vi "Main_08B_Long Wait.vi"() -> ()   [LabVIEW 2025]
uses:
  Cluster_3D Pos.ctl
  41698488-36b5-4046-9fd7-0d51cedffe47.vi
  2bdc9d8d-ae33-491b-9533-2d130997e3b1.vi
  Utility/Universal Utility/TypeDefs_Utility/Cluster_Row-Column.ctl
  9e3f57c0-2ef8-4495-8287-c6a42a5fb955.vi
  Utility/Universal Utility/TypeDefs_Utility/ENUM_4 Directions U-D-L-R.ctl
  Utility/Universal Utility/TypeDefs_Utility/ENUM_8 Directions U-D-L-R.ctl
panel:
  out "Cluster Out":cluster{"Numeric":dbl, "3D Pos":T1, "3D Pos":T1}
  out "Target":i32
  out "Last Size":i32
  out "Numeric":i32
  out "x-y 2":i32
  out "size(s)":i32
  out "x-y":i32
  out "map":map{T1, set{T1}}(c390)
  out "Distances":T2(array[cluster])
  in  "3D Pos":T1
  out "MATCH":bool
  in  "Select Data":enum32{"Example", "Puzzle"}(tab)
  in  "EX Target":u64=25272
  in  "Example":string="162,817,812\n57,618,57\n906,360,560\n592,479,940\n352,342,300\n466,668,158\n542,29,236\n431,825,988\n739,650,466\n52,470,668\n216,146,977\n819,987,18\n117,168,530\n805,96,715\n346,949,466\n970,615,88\n941,993,340\n862,61,35\n984,92,344\n425,690,689"
  in  "Puzzle":string="93612,76992,69452\n4387,60049,8877\n43126,39737,84757\n30167,68987,19789\n92427,53000,95237\n38193,19273,23561\n54992,34511,43980\n11107,44787,52686\n35724,98740,19812\n28016,57751,86155\n93461,77703,78395\n94606,79586,97929\n67878,92289,42528\n38971,54378,98204\n66002,25958,89347\n40281,30990,67294\n25898,31190,14029\n85535,48773,26872\n10128,70597,46452\n68618,23612,85624\n79490,1682,569\n8828,51411,60251\n38583,16324,14091\n10437,63697,61596\n56370,26228,17029\n86199,8063,16493\n20471,66847,99889\n28748,63929,18749\n19248,83995,67615\n333,91140,79303\n59093,5932,49628\n65463,73678,60286\n87559,27061,41247\n424,28274,74202\n85572,19477,32761\n88116,2580,65047\n77302,37669,40015\n7664,30793,17676\n7152,87786,56278\n21754,53651,91511\n19205,97579,71254\n13841,24770,87922\n60676,26132,30482\n10161,34169,42397\n97588,95253,77422\n62674,99068,96065\n3701,85077,92763\n87646,99624,9786\n79480,48455,82469\n85485,88400,12789\n80002,63227,89969\n78922,68131,54845\n11326,3980,91289\n37613,85718,1487\n73551,87391,77749\n18494,53007,56937\n95754,20192,31376\n81009,94209,66866\n89029,86481,28533\n73124,31585,3562\n5647,86375,87389\n17667,62606,81057\n90251,13392,46704\n8922,53813,49554\n90818,72498,63116\n63706,12205,48645\n86075,45959,79136\n8533,98522,94830\n13261,87807,47571\n85512,34571,10686\n70830,45794,26572\n70838,85387,63507\n50514,2902,47654\n97257,76204,25909\n20663,49002,12395\n14787,22089,91493\n9519,20986,37182\n48407,1747,57434\n84550,61928,41891\n27065,7926,77657\n32551,75407,17933\n44728,48491,5096\n28667,99071,90157\n98892,74499,37947\n75619,55121,72752\n36135,20145,68562\n33258,19964,28963\n66217,41845,39708\n32152,82331,42510\n38241,71629,84071\n63645,42508,41998\n18010,23872,31891\n30919,69353,79552\n5249,74361,18723\n51253,57096,69531\n54551,72707,27442\n87816,89043,21120\n43115,24297,19479\n10017,68608,64216\n38916,98813,18429\n53460,96455,10528\n1528,25204,29747\n59806,11528,62206\n84940,6921,98186\n55,22445,44444\n48901,95321,2434\n36897,31163,71124\n733,10092,43971\n95769,23499,86894\n58488,65824,44700\n95535,95053,28430\n62042,11824,48380\n47371,59378,9083\n87851,59391,33276\n71416,91746,80466\n20986,14005,28560\n62877,91310,56300\n44999,12630,89580\n12814,17342,311\n75884,25052,43459\n17057,50968,25293\n8779,78959,17492\n37260,26515,88716\n93030,14321,95804\n51240,43987,47003\n19716,71779,92039\n38192,96721,59996\n3751,16201,26085\n23562,83044,98517\n21091,69932,70564\n17906,89206,87817\n15112,8697,39582\n50853,23583,25901\n4031,58523,46946\n29574,85339,94502\n2159,28840,67804\n64232,21352,6079\n69968,53511,19694\n64707,83228,92602\n68033,91486,5930\n88327,83351,44501\n48616,4913,23373\n64394,88985,96012\n7137,22829,95789\n61147,23131,27577\n9220,73362,24735\n77484,65386,87676\n19406,27628,27294\n36096,5448,80101\n41415,71615,96750\n49579,73718,75680\n51667,75635,2150\n58588,13959,21674\n3301,85861,9573\n39663,82812,63976\n77881,12060,64325\n32096,56047,49426\n87020,81590,63482\n11350,22612,68794\n34318,87015,28581\n88333,30415,72842\n14284,31669,98394\n91299,33003,98512\n50558,25664,87891\n45463,92120,88896\n78928,17342,53217\n85152,36483,90933\n32494,63948,13733\n79538,15123,59524\n13272,69237,88883\n71440,34646,36000\n70887,92196,70756\n86682,49869,59461\n87014,69218,96246\n85096,62446,58342\n47656,42067,94693\n76389,21187,19854\n98808,95119,66355\n56317,4067,58089\n62979,31016,54595\n95574,94910,44555\n92818,89957,30178\n88205,83421,11231\n98025,26158,67351\n34996,37782,12656\n7275,92020,69192\n61755,48578,74891\n91077,87591,13567\n47178,98753,67298\n24890,185,41055\n21656,10424,76098\n36907,5392,33161\n1196,87844,89911\n62084,33566,56665\n66936,13949,44242\n10287,7906,50612\n94242,25001,57410\n75412,1024,29512\n90851,87543,72388\n71747,19001,91980\n22967,72331,12208\n29687,34581,5318\n52323,58423,16852\n86287,3765,36953\n15503,61881,49607\n17730,83252,72329\n32791,46945,9909\n90377,15005,82108\n25088,43430,50889\n30937,67449,69570\n27055,70369,20047\n87796,33912,38981\n61308,25361,93385\n92140,77658,13928\n22619,38036,36441\n66615,58337,19579\n69481,81387,29719\n96348,68719,86050\n50514,639,29192\n75973,520,69761\n82361,79014,99108\n84447,68240,70851\n1603,1169,79818\n17505,5417,49001\n42348,26283,64808\n53052,35593,79353\n29059,44086,34246\n19705,32222,54841\n93505,73226,37229\n88280,88881,65243\n31982,61769,85501\n18942,69659,87848\n48747,77115,64412\n89986,59345,39585\n92036,77473,89017\n54927,93308,13866\n62414,96971,46218\n18054,44880,20543\n18191,85757,79281\n55277,56892,25137\n56722,15970,49886\n65888,61906,88954\n21214,43085,32786\n79619,24041,30679\n22962,60563,90448\n24703,43433,54346\n64964,61426,85237\n81713,50846,23776\n16354,44817,55696\n2131,92987,36071\n24669,58903,97840\n34050,79236,15174\n94757,87186,41770\n60958,81684,89389\n70618,56638,1431\n15922,77068,73670\n84295,36683,59806\n39229,8110,32311\n9957,37073,62331\n58126,91378,50095\n43938,84938,37934\n46924,27412,73996\n78529,43275,80069\n47252,68636,49729\n11419,1422,86133\n32065,82752,94710\n21983,2625,75459\n44369,40437,65291\n45830,99247,97279\n102,35695,58176\n31421,83303,74978\n58281,98901,45492\n106,49263,7938\n14420,24582,44323\n68568,24062,71612\n16050,65447,90641\n7423,8218,42238\n16769,75102,10654\n91505,32646,7194\n94158,35310,78925\n8512,2585,65102\n78362,24338,27827\n61073,96429,1483\n55466,2563,6915\n76849,20355,4244\n23720,88978,85697\n4881,40227,59389\n90297,3954,2223\n71850,58017,89245\n88343,36437,43379\n48699,55848,41462\n87085,80923,41276\n8190,65515,49515\n60930,91345,56495\n775,157,41546\n78449,37056,92044\n25226,37026,8384\n83556,2712,79328\n23265,52246,97851\n84479,51110,40981\n62886,35622,78961\n6523,92713,24122\n25314,54911,73916\n35030,4968,50659\n49041,83519,77623\n15167,26960,96355\n16247,64185,99408\n18474,61281,4969\n13926,31813,16094\n15725,68810,87796\n15464,46735,8813\n13805,10520,11814\n16255,71827,53917\n17481,74068,39973\n1780,6131,70717\n96873,33332,58634\n75700,9121,4357\n15100,24737,23182\n21595,73141,60112\n17623,46752,17930\n966,77550,1372\n23916,5486,61016\n58073,54435,99676\n63398,25454,22034\n11040,78676,89673\n72346,68534,60847\n86865,20480,28605\n10868,89008,17327\n9838,37312,78948\n9843,72664,46882\n25362,3537,55029\n25124,98455,46040\n67429,30617,65289\n50349,91411,86860\n88161,26971,2438\n55654,9333,21695\n21824,81354,24579\n74930,71845,25730\n31018,58510,74464\n63758,31045,74703\n66762,78487,4118\n51908,57077,1574\n36829,63414,74887\n70493,64836,64929\n67420,65219,8818\n67566,17153,99697\n31824,74123,30207\n56502,53943,35115\n17246,97907,98834\n68705,29666,71246\n27724,15999,56550\n60276,22366,14653\n46389,53387,87116\n3235,14486,91436\n49732,63892,87340\n87008,94331,58514\n32145,38609,71845\n64572,18666,90042\n12352,11171,65795\n50884,39309,7436\n72407,18819,32603\n37449,16014,50829\n50516,25437,245\n66137,40543,98203\n28102,29674,6025\n55921,37483,59917\n80575,24800,7675\n44559,17720,81000\n21868,4371,65769\n34785,60526,44642\n5726,52286,31034\n35566,72914,82787\n32070,85672,66017\n19110,93664,19934\n53538,56804,28502\n78852,78651,65871\n99691,96705,52190\n77702,9722,56604\n96505,53849,9751\n85655,28788,96526\n96697,6837,96685\n83162,25825,24329\n48579,28766,854\n88152,9279,65839\n83244,71777,64273\n67540,72397,45717\n33581,56860,73496\n41361,43101,43910\n77896,55800,6729\n11660,9790,41267\n97909,44466,33924\n75949,72557,25770\n2834,8126,65868\n9551,65106,23021\n16497,40985,62744\n2394,85493,15918\n13869,86996,34945\n7314,71681,76769\n8314,17091,51115\n21559,78084,38617\n23289,65563,77867\n56384,16752,25872\n73173,27198,18275\n14487,89322,53052\n43042,74199,19715\n79730,3967,66686\n49193,63676,8674\n75653,71020,71125\n76566,82061,60310\n62574,19011,34913\n7784,78818,4837\n96246,64285,64844\n28376,38429,5472\n29362,65551,35253\n86883,51698,98020\n24309,19686,76751\n79120,49475,86875\n21875,26909,80928\n26647,97704,47621\n81672,4744,85242\n1531,59200,59569\n32899,26845,37534\n44049,35082,85646\n76568,75911,25179\n8965,84562,95316\n84091,11217,36912\n75391,5840,53123\n65257,29963,25808\n37711,89932,64085\n58313,77455,73975\n50094,87928,18598\n5972,26111,44908\n18007,13342,78943\n76931,50984,47834\n21067,16782,67472\n15702,16241,74410\n87250,79827,72823\n39856,29885,87881\n63010,34722,55942\n66094,53196,60158\n66103,13376,41069\n50817,73301,75220\n92689,896,59366\n25127,93940,535\n26486,26180,69703\n30551,201,44121\n57951,59180,74903\n81875,39479,66376\n75608,64370,34924\n65874,46991,20843\n64546,80899,48722\n53139,81240,60912\n6408,95126,99539\n60382,32038,26842\n51897,69343,23769\n12903,64987,23678\n89816,57639,2794\n91943,17916,68132\n17058,47490,53424\n63508,59639,78981\n24149,76305,83221\n59786,97124,35477\n7654,4401,5943\n65324,87395,56976\n1254,59660,42700\n28520,51382,13607\n32395,72384,24714\n98919,51493,35815\n85861,23706,42361\n73727,19357,9192\n56244,61066,88568\n69022,93334,95441\n45135,78907,67376\n71905,21859,53682\n76240,18122,86744\n96451,36880,58724\n69809,81170,43323\n91766,30035,70211\n94430,93928,35098\n36019,86391,62142\n29610,48551,78565\n61687,61798,44674\n83243,280,87775\n12879,46004,26625\n35774,96599,27266\n54000,69437,46041\n53659,5289,64037\n74733,24414,37294\n97525,10350,59878\n27775,49801,65616\n1659,48519,9189\n4829,84196,28561\n60895,93831,21468\n61573,4274,9651\n98125,85369,35792\n52818,38024,65559\n84495,67225,93469\n32787,83707,84703\n62567,37936,64206\n94030,89183,13432\n13072,95484,27690\n23734,31846,65035\n92988,93579,66115\n78711,53315,59155\n54913,63455,29728\n62483,46401,60745\n20788,21695,50675\n42551,84909,54997\n852,73770,55668\n10942,89879,3343\n88911,85683,58125\n8888,4740,64248\n61357,52361,84989\n59211,31184,957\n68198,89759,1696\n66912,82567,26659\n63452,49304,14117\n55562,86015,61863\n96167,90245,35196\n83946,59012,8249\n83464,21575,9933\n20029,49554,45712\n45708,6745,4125\n33357,87835,35297\n86141,60426,87671\n48011,2841,34713\n70487,20646,44208\n52285,77621,30036\n59856,65624,60884\n92153,97045,59609\n77434,44541,28160\n99278,3474,2582\n44670,87341,16251\n16908,23106,9882\n3599,76235,82771\n55003,24153,14048\n31115,24573,17690\n93842,2483,76226\n19930,22308,31182\n97987,68482,5762\n97753,36572,53143\n56946,55429,42606\n4114,37864,84931\n20033,73108,2340\n63076,45812,25089\n68562,32600,71420\n60368,97785,65980\n5445,48961,97781\n58844,71797,9869\n77623,23298,19643\n68939,99057,77762\n47164,99255,46365\n17824,73903,89733\n44488,67436,26816\n10626,19619,37213\n78525,91601,18913\n87482,17097,99480\n89825,9580,23005\n81850,94513,95910\n58710,20827,82163\n84830,30431,42014\n19885,2222,91325\n29036,50455,10625\n14579,68427,88723\n46506,57905,65480\n25501,25015,65137\n34126,92382,12760\n42990,35933,69002\n76547,12396,70799\n27867,68712,54134\n58345,5062,87052\n51715,80934,28246\n74189,23723,30837\n98243,92321,40231\n42351,5969,15336\n29632,29612,22258\n31543,13513,60004\n51272,2995,7475\n96993,16572,7646\n8241,53230,7612\n20137,54640,20893\n59566,7551,18524\n40530,53994,15411\n6874,38747,96386\n60096,17731,1885\n21358,47158,57995\n48040,27043,44231\n90293,31220,5002\n87034,57231,1922\n47580,56506,51457\n21645,43851,33340\n50203,31461,99819\n29924,64669,80294\n48937,97069,87025\n56459,76682,90702\n39922,84072,64788\n56086,33603,60174\n57079,95782,95195\n93093,10317,85610\n4553,96124,53294\n70238,97923,20386\n76705,37902,51495\n18376,89053,50239\n43721,95653,31712\n97543,903,77076\n63809,98240,32449\n19598,27244,51311\n58861,93737,38995\n46246,70148,17082\n44972,2348,38868\n6647,2768,40251\n59453,62399,43434\n27211,23165,55801\n31210,4420,40809\n67954,89265,21307\n38157,58874,65993\n17047,12135,98851\n65082,3379,10087\n14995,71193,92046\n85554,218,47029\n52869,68400,61476\n15245,89469,36381\n1523,36104,35383\n81169,162,47941\n36480,61750,92719\n9137,30924,39406\n4656,6959,26256\n94128,50715,27623\n17165,55297,17490\n93520,76418,8404\n31533,5640,75764\n3115,47128,2667\n70908,20297,33409\n91667,83564,10987\n78738,79975,79614\n98601,79197,63374\n22489,6709,19769\n3661,48606,4034\n62587,69293,92052\n31430,11646,58643\n80493,23478,52020\n76806,36625,61325\n52254,77479,79176\n89958,48556,1961\n5928,19241,90408\n71968,16233,65908\n49587,3396,51724\n15836,73105,68814\n87142,20107,78921\n19987,26258,32877\n47137,5614,19848\n88710,50130,58513\n12385,24867,62286\n88852,6913,44817\n21656,66145,71816\n13390,54530,54277\n557,41725,27372\n30345,90380,49797\n95541,28277,63610\n15296,61358,32017\n96483,11065,83679\n31183,4570,40265\n69674,28710,2052\n21841,48430,57641\n20947,65038,17338\n39281,94409,83606\n53035,53090,82421\n22343,46641,9487\n37999,11874,10825\n28891,74850,94585\n87115,56628,33382\n14619,74286,45544\n39133,78470,91243\n42199,76781,37404\n64919,33295,42593\n37280,99390,75546\n99850,21071,86687\n12561,14737,51205\n82463,8628,46379\n66413,6177,22765\n64129,76197,71439\n42257,60362,76910\n88537,67489,68630\n38,59181,27553\n18122,55369,49886\n36309,97303,40682\n51847,12862,36119\n63247,24005,69216\n79104,66384,54736\n56017,25641,12457\n44064,88259,80773\n29737,522,94568\n45720,48619,8513\n32824,94363,98444\n66637,42496,26435\n2012,34374,99911\n63462,34544,82946\n60906,96191,27861\n889,8875,96367\n20701,850,32374\n48614,31194,51795\n81219,24377,57375\n80635,53805,27351\n73080,55463,50428\n63827,57808,55144\n51107,90419,84912\n18717,94186,31613\n49169,44719,10443\n39615,75279,12347\n11964,45685,47665\n30923,15472,65080\n5,94188,54596\n14379,13017,44646\n77743,60302,80107\n9067,49328,81390\n3402,88018,48284\n8590,94702,4002\n53713,46872,45856\n88918,2415,28532\n46287,21781,14851\n29324,9071,81874\n96983,92983,94390\n26328,6604,67828\n15607,19849,9427\n3777,80212,69260\n66785,89681,58809\n47599,81474,12698\n19680,28606,58721\n84565,96029,9266\n6807,28162,25245\n37858,37187,33146\n74215,20317,21602\n36577,27799,76382\n7377,35371,6580\n7134,79656,97584\n9214,10648,27402\n71686,59728,6298\n19675,43121,23335\n59814,19764,9046\n29503,20036,61270\n21728,78643,8960\n25275,32799,80768\n44283,98410,81536\n79332,8520,54150\n45424,1453,21479\n94250,78055,73228\n79489,63243,23534\n74398,21497,19692\n26191,34756,90513\n15902,65731,1896\n20962,19514,89850\n19048,85210,61442\n95612,27282,33774\n34539,17019,59356\n15886,4956,6561\n85554,43774,56068\n83399,44069,83268\n24967,47996,80688\n4261,39672,3487\n1927,90969,36407\n56341,31181,98469\n59463,4377,44429\n98081,89435,28196\n47337,146,41069\n34676,62991,93667\n40830,18095,3895\n33969,71800,98522\n55019,22833,33982\n18690,49810,11880\n49895,63070,57918\n65670,75982,47329\n86680,2893,7573\n5834,19741,15335\n84314,61210,54625\n38876,95177,55552\n93526,89293,47002\n17120,25610,64975\n86677,14247,90832\n22687,49968,65263\n33489,61528,47384\n24128,84568,80402\n32790,66977,67469\n31024,33923,53791\n70747,28366,81550\n50357,79826,64276\n19955,61357,45034\n76265,15144,70455\n33272,27568,76909\n84054,28474,14905\n81452,3560,64204\n2995,78946,98322\n56789,88645,28228\n55217,64868,79116\n53070,48551,745\n68657,22409,8500\n19161,61390,32918\n90698,82905,97853\n5723,32433,63684\n34840,90469,60825\n56921,24222,16744\n29618,35579,65053\n13778,57959,19521\n25635,79962,26765\n11711,67792,70774\n25724,32520,56341\n60970,2201,40013\n12431,49332,27831\n42375,12958,13514\n370,13074,49841\n91947,38771,98238\n26114,98967,4911\n36520,71551,49807\n12961,85927,32810\n41687,29135,297\n13647,65415,53114\n14884,74124,94717\n55608,71741,17940\n93046,29518,14342\n74408,38008,7480\n28472,49579,78045\n30644,35566,90190\n1309,18579,30254\n97408,9395,71712\n37963,73038,17907\n9746,1554,53649\n17312,72556,34581\n30416,98565,14025\n67271,28750,53687\n89089,94797,85638\n5584,98314,42396\n27573,12427,67217\n9685,20315,45779\n5783,89296,50119\n7395,30,59651\n59962,33958,16528\n86075,23394,31491\n63546,81157,1594\n79123,11575,47557\n18756,75540,70443\n72748,68961,58742\n81525,73484,89742\n21011,49906,40935\n73943,81252,41073\n70776,51604,32224\n80561,65802,5922\n51505,27172,13520\n26382,9698,48756\n2966,37811,41624\n64790,93568,62536\n11099,33411,14293\n82091,74600,4338\n65085,60858,10082\n10035,21650,50785\n63805,33377,24475\n21382,39590,34505\n97345,3372,97760\n70419,80414,3046\n69513,27185,34584\n45800,92516,45439\n35481,65400,79823\n29374,6114,11941\n14303,82901,68795\n41717,69307,75349\n56279,66633,83524\n1428,66470,56206\n12553,6733,20622\n86659,41648,61379\n52033,36683,50080\n86318,10074,13631\n45812,45986,76341\n15567,44527,88436\n8379,59777,5722\n32237,18036,35978\n93679,5115,61935\n29374,36888,40254\n40168,44291,77176\n35156,24957,90910\n41864,98051,46439\n55645,27893,16675\n59670,98073,46841\n22314,81305,24733\n61273,22761,81192\n11266,14830,95245\n22284,40607,66310\n64598,79802,15581\n28610,12550,19851\n91295,60386,36743\n49527,66039,86751\n88255,50623,11696\n36872,95176,1262\n16382,84203,28357\n62874,36513,89144\n80390,41087,3818\n28934,77608,84891\n50028,68867,41659\n97663,86772,45290\n17334,17423,10170\n86813,9459,20678\n7354,26123,3088\n34601,83872,75235\n82487,85716,87179\n74872,55822,94773\n67775,20758,74726\n1637,23257,96839\n70086,38606,11329\n37333,4381,74577\n96787,23125,65361\n16240,10806,28282\n45777,86620,58681\n36901,96007,61808\n59798,96493,52712\n14613,28066,56986\n22873,73388,8548\n83152,66623,6706\n89253,53707,70248\n63732,55857,79585\n33389,99411,36126\n30138,88565,73193\n33385,56862,9781\n79007,32407,2149\n20654,78581,52328\n45915,25675,21594\n7534,54164,58394\n33997,15513,56367\n84919,21671,57105\n64175,41950,67051\n24936,26061,83072\n35451,62404,35874\n88295,14526,66310\n51289,61271,70041\n67716,12185,49570\n93006,31081,47748\n48016,50057,50060\n6631,7960,36378\n78124,51652,45315\n84586,11610,77166\n59601,95521,21125\n38937,84911,35085\n39499,37095,46732\n93972,71312,67295\n8864,15288,17706\n23399,15100,53520\n72344,82783,41899\n45766,36673,75853\n19760,87756,29939\n25227,74446,3738\n14331,10331,24476\n76223,50493,23898\n18356,62271,85875\n53608,20015,32714\n83392,67440,55013\n68424,46958,45601\n19431,26823,16321\n38932,60197,69781\n40297,68548,88034\n2968,29193,15002\n92059,26056,54737\n54184,66310,1075\n95784,57910,81595\n75602,59936,8544\n72249,27430,48332\n55862,41522,43934\n414,95763,96341\n33017,8463,42855\n51476,85018,43369\n60252,91356,87437\n36938,80351,62343\n84358,62436,51394\n88131,91800,50091\n75336,70492,41687\n91456,89983,51215\n17937,73395,45724\n80843,13138,64230\n49657,60368,32741\n56682,33989,9564\n73621,44474,4935\n63853,84785,75892\n29391,81042,4538\n31349,63646,21745\n55645,20057,48322\n51551,58220,79615\n21562,48950,99930\n1841,5768,17379\n40557,47811,27557\n20849,49275,68348\n44177,45015,99771\n15266,88740,35835\n22445,30430,59975\n68881,21591,89341\n76719,38478,66227\n73301,82485,38111\n8828,57991,18536\n94665,49942,59110\n15225,58083,66890\n29518,68804,75755\n50130,82904,45313\n63183,52674,91427\n97487,63178,89472\n3968,12975,47549\n22818,54619,79778"
  in  "Puzzle Target":u64=3767453340
  out "Answer":u64
  # "18446744073182037660 Is Too HIGH"
  # "15980 Too LOW"
  # "Product of the X Positions that connected\nall boxes"
  # "Product of the X Positions that connected\nall boxes"
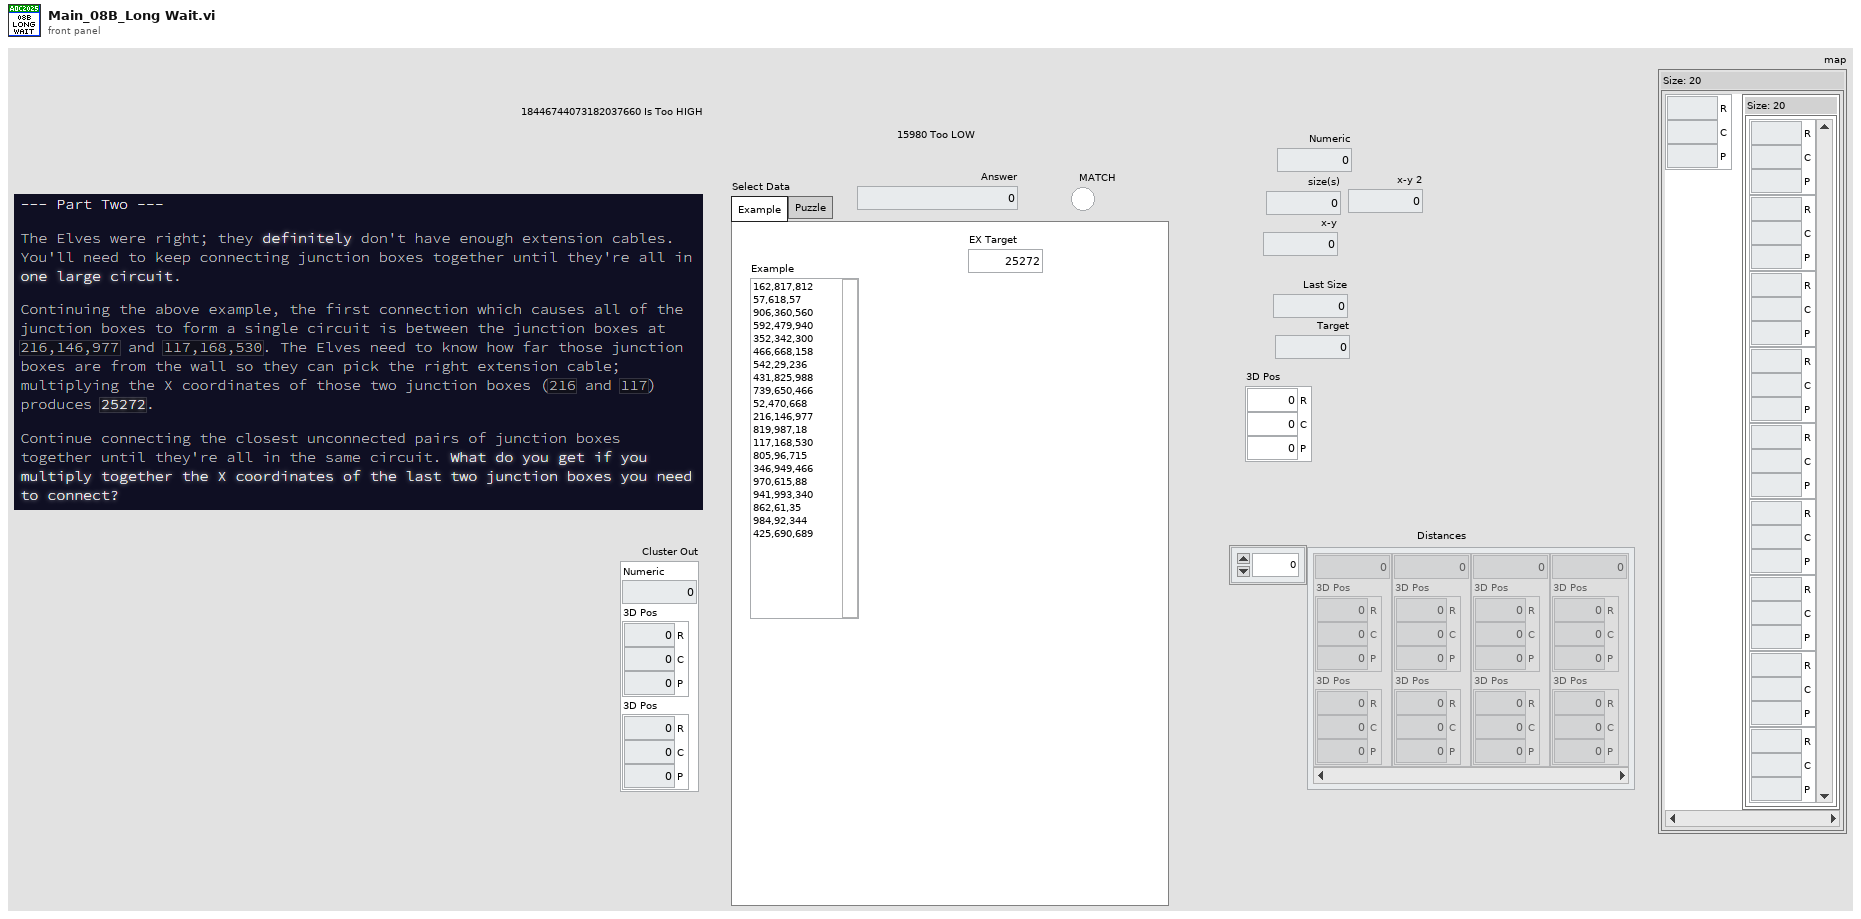
[diagram p1: front panel]
types:
  T1 = typedef "Cluster_3D Pos.ctl" = cluster{"R":i32, "C":i32, "P":i32}
  T2 = cluster{"Numeric":dbl, "3D Pos":T1, "3D Pos":T1}[]
  T3 = typedef "ENUM_8 Directions U-D-L-R.ctl" = enum16{"Up;-1,0", "Up-Right;-1,1", "Right;0,1", "Down-Right;1,1", "Down;1,0", "Down-Left;1,-1", "Left;0,-1", "Up-Left;-1,-1"}
  T4 = typedef "ENUM_4 Directions U-D-L-R.ctl" = enum16{"Up;-1,0", "Right;0,1", "Down;1,0", "Left;0,-1"}
  T5 = typedef "Cluster_Row-Column.ctl" = cluster{"R":i32, "C":i32}
  T6 = typedef "Cluster_Distance Data.ctl" = cluster{"Distance":dbl, "StartPos":T1, "End Pos":T1}
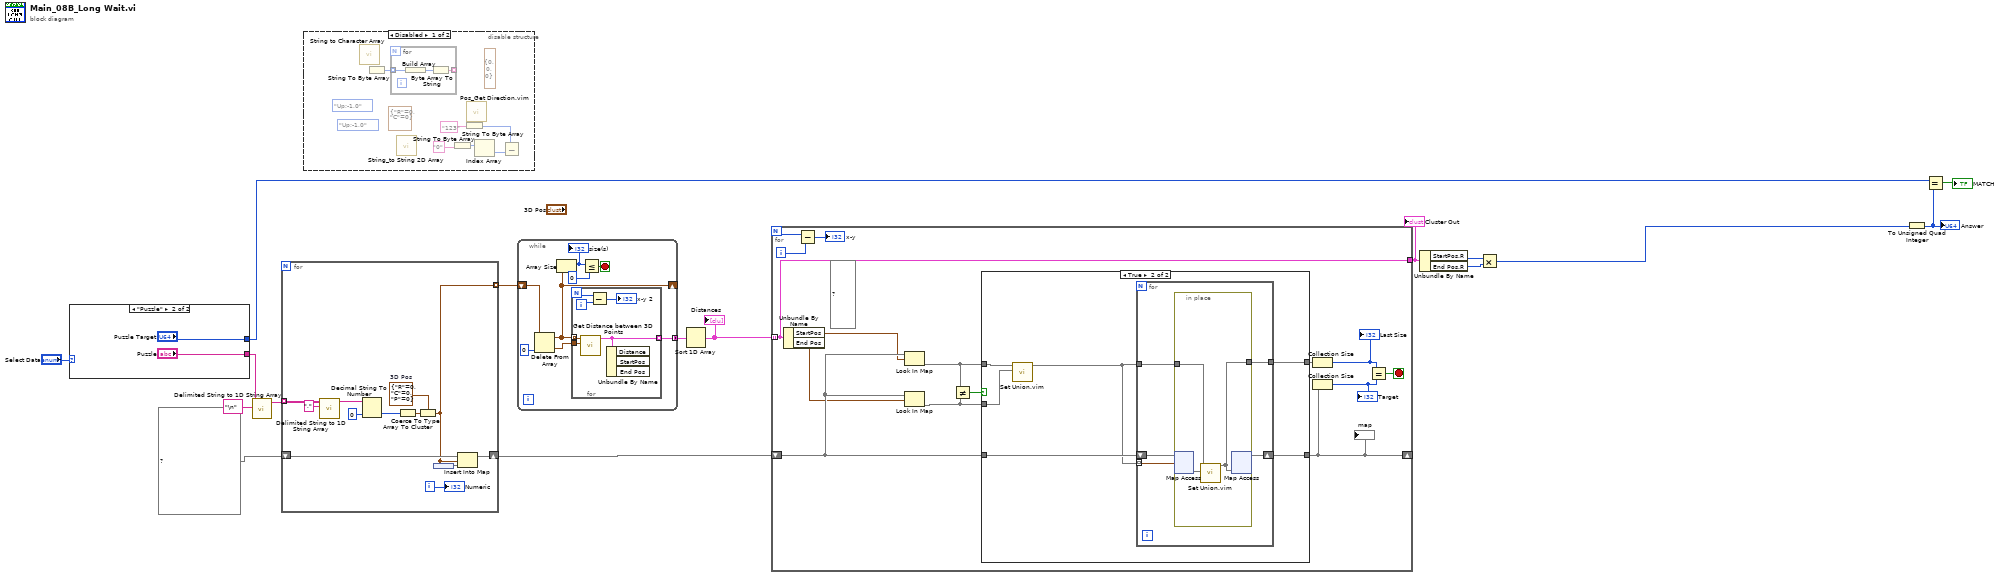
[diagram p0: block diagram]
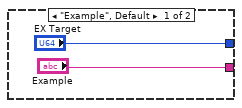
[diagram p3: hidden frame]
diagram:
  n1 = case shown="\"Puzzle\"" "Select Data" {
    tunnel: ["Example" "Puzzle"] -> w14
    tunnel: ["EX Target" "Puzzle Target"] -> w11
    frame "Example", Default {
    }
    frame "Puzzle" {
    }
  }
  n2 = call <vilib>:"Delimited String to 1D String Array.vi"("delimiter"="\n" ("delimiter (Tab)"), "delimited string"=w14) -> ("string array"=w15:string[])  [unwired: 9 in]
  n3 = for {
    tunnel: w15 -> [w32] mode=indexing
    tunnel: [w23] -> w9 mode=indexing
    shift-right: [w24] -> w5
    shift-left: map{T1, set{T1}} {} ("map") -> [w25]
    i -> [w21]
    w26 = T1 {"R"=0, "C"=0, "P"=0}  # 3D Pos
    n4 = call <vilib>:"Delimited String to 1D String Array.vi"("delimiter"=",", "delimited string"=w32) -> ("string array"=w30:string[])  [unwired: 9 in]
    n5 = Decimal String To Number(string=w30, default (0L)=u64 0 ("default (0 I32)")) -> (number=w28:u64[])  [unwired: 1 in, 1 out]
    n6 = Array To Cluster(array=w28) -> (cluster=w27:cluster{"[0]":u64, "[1]":u64, "[2]":u64})
    n7 = Coerce To Type(0:w27, 1:w26) -> (2:w23:T1)
    n8 = node(w23) -> (w22:set{T1})
    n9 = Insert Into Map(map in=w25, key=w23, value=w22) -> (map out=w24:map{T1, set{T1}})  [unwired: 2 out]
    "Numeric" <- w21
  }
  n10 = disable-structure shown="Disabled" {
    frame Disabled {
      (unwired) T1 {"R"=0, "C"=0, "P"=0} ("Position")
      (unwired) ENUM_8_Directions_U-D-L-R."Up;-1,0" ("Direction 8")
      (unwired) ENUM_4_Directions_U-D-L-R."Up;-1,0" ("Direction")
      (unwired) T5 {"R"=0, "C"=0} ("Position")
      n11 = call "String to Character Array.vi"() -> ()  [unwired: 1 in, 1 out]
      n12 = String To Byte Array() -> (unsigned byte array=w33:u8[])  [unwired: 1 in]
      n13 = for {
        tunnel: w33 -> [w41] mode=indexing
        tunnel: [w39] -> _ mode=indexing
        n14 = Build Array(w41) -> (w40:u8[])
        n15 = Byte Array To String(unsigned byte array=w40) -> (string=w39:string)
      }
      n16 = call "String_to String 2D Array.vi"() -> ()  [unwired: 11 in, 1 out]
      n17 = String To Byte Array(string="0") -> (unsigned byte array=w36:u8[])
      n18 = String To Byte Array(string="123") -> (unsigned byte array=w34:u8[])
      n19 = call "Pos_Get Direction.vim"() -> ()  [unwired: 11 in, 1 out]
      n20 = Index Array(array=w36) -> (element=w35:u8)  [unwired: 1 in]
      n21 = Subtract(x=w34, y=w35) -> ()  [unwired: 1 out]
    }
    frame Enabled {
    }
  }
  n22 = while {
    shift-right: [w45] -> _
    shift-left: w9 -> [w49]
    tunnel: [w46] -> w8 mode=concatenating
    stop <- w42 stop-if-true
    n23 = Delete From Array(array=w49, index=0) -> (deleted portion=w47:T1, array with subset deleted=w45:T1[])  [unwired: 1 in]
    n24 = Array Size(array=w45) -> (size(s)=w44:i32)
    "size(s)" <- w44
    n25 = for {
      N -> [w53]
      tunnel: w45 -> [w54] mode=indexing
      tunnel: w47 -> [w55]
      tunnel: [w50] -> w46 mode=indexing
      i -> [w52]
      n26 = call "Get Distance between 3D Points.vi"(10:"3D Pos"=w55, 11:"3D Pos"=w54) -> ("Distance Data Out"=w50:T6)  [unwired: 9 in]
      n27 = Subtract(x=w53, y=w52) -> (x-y=→"x-y 2":i32)
      n28 = Unbundle By Name(w50) -> ()  [unwired: 3 out]
    }
    n29 = Less Or Equal?(x=w44, y=0) -> (x <= y?=w42:bool)
  }
  n30 = Sort 1D Array(array=w8) -> (sorted array=w7:T6[])
  "Distances" <- w7
  n31 = for {
    N -> [w70]
    tunnel: w7 -> [w64] mode=indexing
    shift-right: [w57] -> _
    shift-left: w5 -> [w63]
    tunnel: [w64] -> w4
    i -> [w69]
    stop <- w65 stop-if-true
    (unwired) set{T1} {} ("value")
    n32 = Unbundle By Name(w64) -> ("StartPos"=w61:T1, "End Pos"=w62:T1)
    n33 = Subtract(x=w70, y=w69) -> (x-y=→"x-y":i32)
    n34 = Look In Map(map=w63, key=w61) -> (value=w60:set{T1})  [unwired: 1 in, 1 out]
    n35 = Look In Map(map=w63, key=w62) -> (value=w59:set{T1})  [unwired: 1 in, 1 out]
    n36 = Not Equal?(x=w60, y=w59) -> (x != y?=w58:bool)
    n37 = case shown="True" w58 {
      tunnel: [w72 w78] -> w57
      tunnel: w63 -> [w72 w77]
      tunnel: w59 -> [_ w76]
      tunnel: w60 -> [w71 w75]
      tunnel: [w71 w73] -> w56
      frame False {
      }
      frame True {
        n38 = call "Set Union.vim"("set 2"=w76, "set 1"=w75) -> ("union"=w74:set{T1})  [unwired: 9 in]
        n39 = for {
          tunnel: w74 -> [w82] mode=indexing
          shift-right: [w80] -> w78
          shift-left: w77 -> [w83]
          tunnel: w74 -> [w81]
          tunnel: [w79] -> w73
          n40 = in-place {
            in-place-border: w81 -> [w86]
            in-place-border: [w84] -> w79
            n41 = in-place-map #1(w83, w82) -> (w85:set{T1})  [unwired: 1 in, 1 out]
            n42 = call "Set Union.vim"("set 2"=w85, "set 1"=w86) -> ("union"=w84:set{T1})  [unwired: 9 in]
            n43 = in-place-map #1(w84) -> (w80:map{T1, set{T1}})  [unwired: 1 in, 2 out]
          }
        }
      }
    }
    "map" <- w57
    n44 = Collection Size(1:w56) -> (0:w67:i32)
    "Last Size" <- w67
    n45 = Collection Size(1:w57) -> (0:w66:i32)
    "Target" <- w66
    n46 = Equal?(x=w67, y=w66) -> (x = y?=w65:bool)
  }
  "Cluster Out" <- w4
  n47 = Unbundle By Name(w4) -> ("StartPos.R"=w3:i32, "End Pos.R"=w2:i32)
  n48 = Multiply(x=w3, y=w2) -> (x*y=w1:i32)
  n49 = To Unsigned Quad Integer(1:w1) -> (0:w10:u64)
  "Answer" <- w10
  n50 = Equal?(x=w11, y=w10) -> (x = y?=→"MATCH":bool)
